vi "Input Dynamic Data Types.vi"(1 "Data Types":T2(array[cluster]), 2 "Data Names&Defaults":string[][](array[string])) -> (0 "Data Names&Data":string[][](array[string]))   [LabVIEW 2016, in "TSPopup.lvlib"]
doc: "Demo showing dynamically changing data types and working with a tree.\n\nType Sensitive Popup \nCopyright © 2007, J. David Saunders\nAll rights reserved."
uses:
  <userlib>/TSPopup/TSPopup.lvlib
  <userlib>/TSPopup/TSPopup.Popup Cluster.ctl
  <userlib>/TSPopup/TSPopup.lvclass
  <userlib>/TSPopup/TSPopup.Popup Call Parameters.ctl
  <userlib>/TSPopup/TSPopup.Data Type.ctl
panel:
  in  "Popups":T1 {"Boolean" items=["False", "True"]; "Ring" items=["X", "Y", "Z", "R1", "R3"]}
  in  "Cancel Button":bool
  in  "OK Button":bool
  in  "Data List":i32(listbox)
  # "Type Sensitive Popup \nCopyright © 2007, J. David Saunders\nAll rights reserved."
  # "Type Sensitive\nPopup"
  # "Boolean Colors"
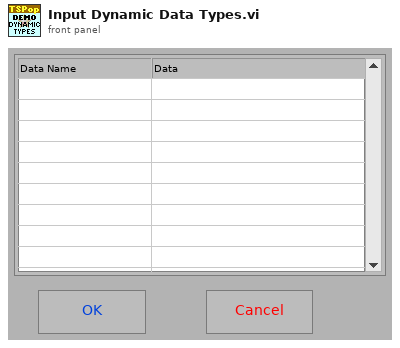
[diagram p1: front panel]
types:
  T1 = typedef "TSPopup.lvlib/TSPopup.lvclass/TSPopup.Popup Cluster.ctl" = cluster{"Unknown":bool, "Unknown 2":bool, "String":string, "Integer":i32, "Float":dbl, "Color":u32, "Boolean":u32, "Ring":u32, "Captioned String":cluster{"String":string, "OK":bool, "Cancel":bool}, "Captioned Integer":cluster{"First":i32, "OK":bool, "Cancel":bool}, "Boolean Colors":cluster{"False":cluster{"FG":u32, "BG":u32}, "True":cluster{"FG":u32, "BG":u32}, "T  to  F":cluster{"FG":u32, "BG":u32}, "F  to  T":cluster{"FG":u32, "BG":u32}, "OK":bool, "Cancel":bool}, "2-Int Cluster":cluster{"First":i32, "Second":i32, "OK":bool, "Cancel":bool}, "4-Int Cluster":cluster{"First":i32, "Second":i32, "Third":i32, "Fourth":i32, "OK":bool, "Cancel":bool}, "check":bool}
  T2 = cluster{"Data Type":string, "Caption/Ring Strings":string[]}[]
  T3 = typedef "TSPopup.lvlib/TSPopup.lvclass/TSPopup.Popup Call Parameters.ctl" = cluster{"Prop Type":T4, "Initial Value":variant, "Caption Strings":string[], "Ring Strings":string[], "Cell Rect":cluster{"left":i16, "top":i16, "right":i16, "bottom":i16}, "Mouse Coords":cluster{"x":i16, "y":i16}, "Call Data":variant}
  T4 = typedef "TSPopup.lvlib/TSPopup.lvclass/TSPopup.Data Type.ctl" = enum16{"Unkown", "NO POPUP", "String", "Integer", "Float", "Color", "Boolean", "Ring", "Captioned String", "Captioned Integer", "Button Color", "2 Int Cluster", "4 Int Cluster", "check"}
  T5 = typedef "LVPoint32TypeDef.ctl" = cluster{"Horizontal":i32, "Vertical":i32}
  T6 = typedef "TSPopup.lvlib/TSPopup.lvclass/TSPopup.Grid.Cell Info.ctl" = cluster{"Tag":string, "Row":i32, "Column":i32, "In Symbol?":bool, "In Data?":bool, "Cell String":string, "Ctl Refnum":refnum<vi>, "Prop Type":T4, "Ring Strings":string[]}
  T7 = cluster{"Data Type":string, "Caption/Ring Strings":string[]}
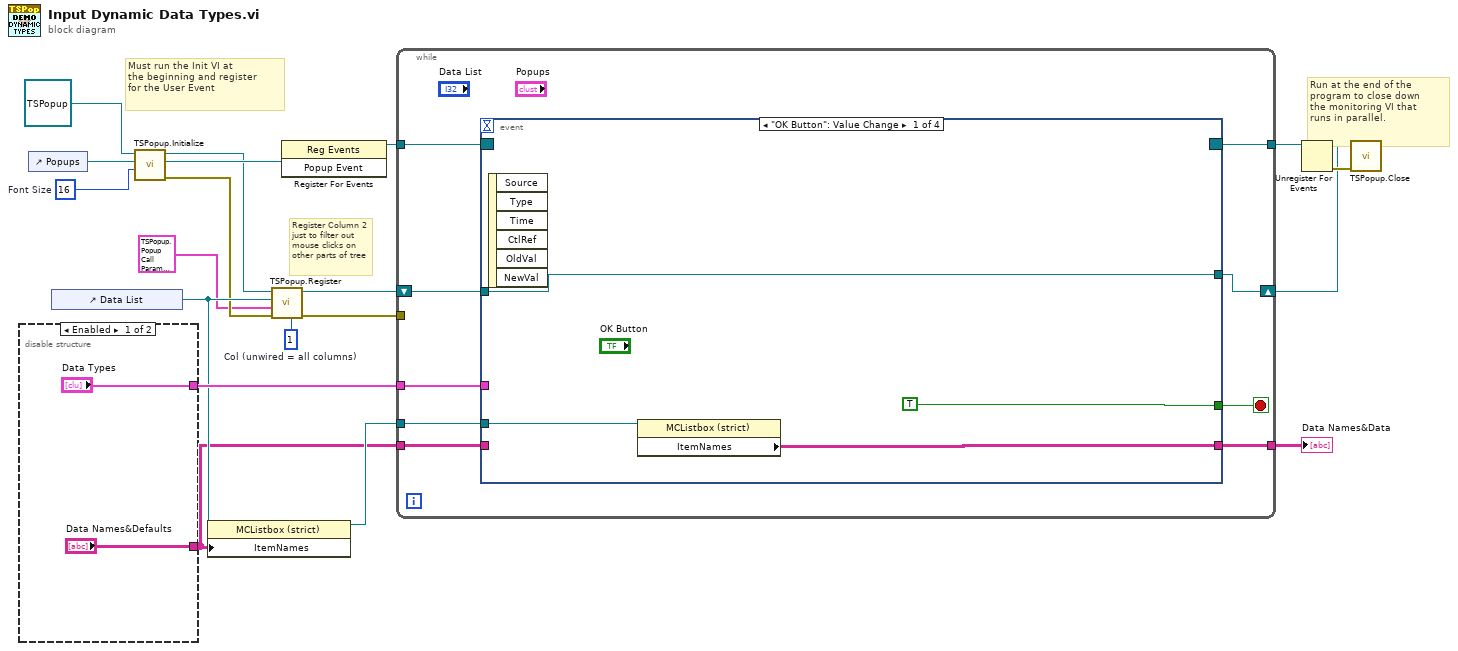
[diagram p0: block diagram]
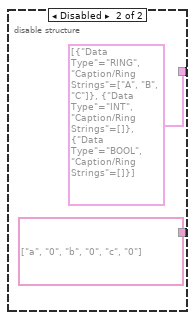
[diagram p2: hidden frame]
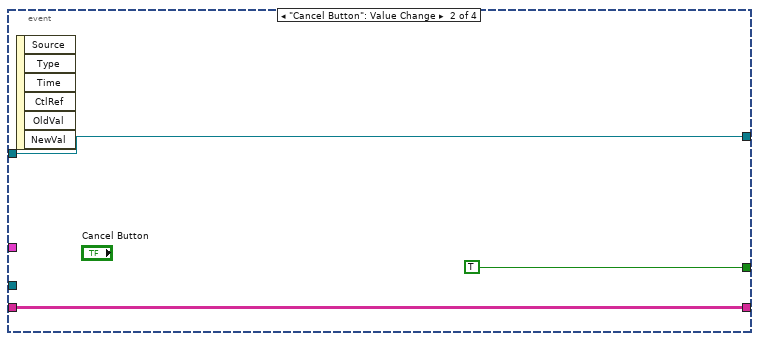
[diagram p3: hidden frame]
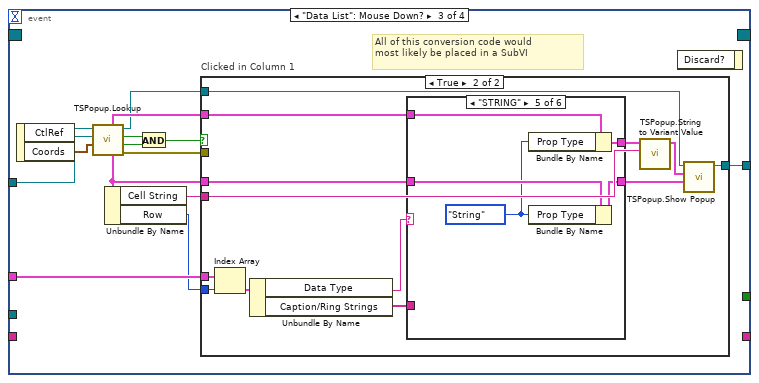
[diagram p4: hidden frame]
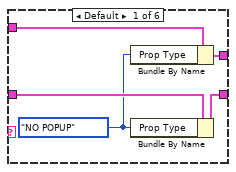
[diagram p6: hidden frame]
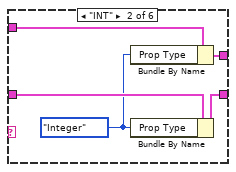
[diagram p7: hidden frame]
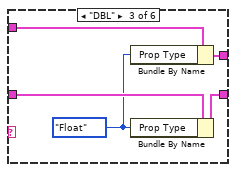
[diagram p8: hidden frame]
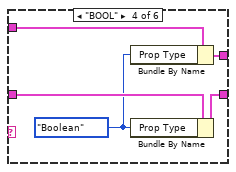
[diagram p9: hidden frame]
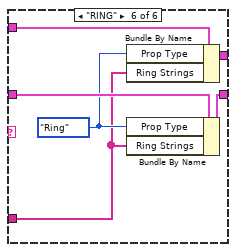
[diagram p10: hidden frame]
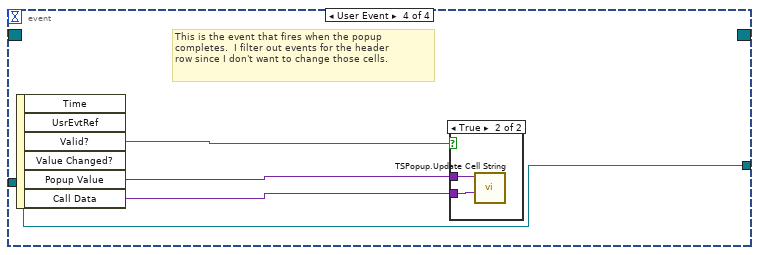
[diagram p11: hidden frame]
diagram:
  w10 = 1  # Col (unwired = all columns)
  w14 = u32 16  # Font Size
  # "Register Column 2\njust to filter out\nmouse clicks on\nother parts of tree"
  # "Run at the end of the\nprogram to close down\nthe monitoring VI that\nruns in parallel."
  # "Must run the Init VI at\nthe beginning and register\nfor the User Event"
  n1 = disable-structure shown="Enabled" {
    disable-tunnel: ["Data Types" T2 [{"Data Type"="RING", "Caption/Ring Strings"=["A", "B", "C"]}, {"Data Type"="INT", "Caption/Ring Strings"=[]}, {"Data Type"="BOOL", "Caption/Ring Strings"=[]}] ("Data Types")] -> w16
    disable-tunnel: ["Data Names&Defaults" string[][] [["a", "0"], ["b", "0"], ["c", "0"]] ("Data Names&Defaults")] -> w1
    frame Enabled {
    }
    frame Disabled {
    }
  }
  n2 = control-ref of="Popups"() -> (w4:refnum<vi>)
  n3 = control-ref of="Data List"() -> (w11:refnum<vi>)
  n4 = call <userlib>:"TSPopup.Initialize.vi"("Font Size"=w14, "Popup Cluster Ref"=w4, "TSPopup in"=refnum<class "TSPopup.lvclass"> refnum ("TSPopup.lvclass")) -> ("error out"=w8:errorcluster, "Popup Event"=w13:refnum<user-event>, "TSPopup out"=w12:refnum<class "TSPopup.lvclass">)  [unwired: 6 in]
  n5 = property class="MCListbox (strict)"(reference=w11, "ItemNames"=w1) -> (reference out=w3:refnum<vi>)  [unwired: 1 in, 1 out]
  n6 = call <userlib>:"TSPopup.Register.vi"("Col (unwired = all columns)"=w10, "error in (no error)"=w8, "Parameters"=T3 {"Prop Type"=enum."String", "Initial Value"=variant, "Caption Strings"=[], "Ring Strings"=[], "Cell Rect"={"left"=0, "top"=0, "right"=0, "bottom"=0}, "Mouse Coords"={"x"=0, "y"=0}, "Call Data"=variant}, "Ctl Refnum"=w11, "TSPopup in"=w12) -> ("error out"=w9:errorcluster, "TSPopup out"=w7:refnum<class "TSPopup.lvclass">)  [unwired: 4 in, 1 out]
  n7 = register-events(w13) -> (reference out=w19:refnum<event-registration>)  [unwired: 2 in, 1 out]
  n8 = while {
    tunnel: w19 -> [w32]
    tunnel: [w31] -> w18
    tunnel: w16 -> [w29]
    tunnel: w9 -> [_]
    shift-right: [w27] -> w6
    shift-left: w7 -> [w28]
    tunnel: w3 -> [w26]
    tunnel: [w25] -> w2
    tunnel: w1 -> [w24]
    stop <- w30 stop-if-true
    n9 = event shown="[0] \"OK Button\": Value Change" {
      selector: w32 -> [_ _ _ _]
      dyn-events: [_ _ _ _] -> w31
      timeout: _ -> [_ _ _ _]
      tunnel: [TRUE TRUE _ _] -> w30
      tunnel: w29 -> [_ _ w51 _]
      tunnel: w28 -> [w35 w38 w42 w99]
      tunnel: [w35 w38 w40 w99] -> w27
      tunnel: w26 -> [w34 _ _ _]
      tunnel: [w33 w37 _ _] -> w25
      tunnel: w24 -> [_ w37 _ _]
      event "OK Button": Value Change {
        n10 = event-data() -> ()  [unwired: 1 in, 6 out]
        n11 = property class="MCListbox (strict)"(reference=w34) -> ("ItemNames"=w33:string[][])  [unwired: 1 in, 2 out]
      }
      event "Cancel Button": Value Change {
        n12 = event-data() -> ()  [unwired: 1 in, 6 out]
      }
      event "Data List": Mouse Down? {
        # "All of this conversion code would\nmost likely be placed in a SubVI"
        n13 = event-data() -> ("CtlRef"=w49:refnum<vi>, "Coords"=w48:T5)  [unwired: 1 in]
        n14 = call <userlib>:"TSPopup.Lookup.vi"("Point"=w48, "Ctl Refnum"=w49, "TSPopup in"=w42) -> ("error out"=w44:errorcluster, "In Bounds?"=w45:bool, "Found"=w46:bool, "TSPopup out"=w41:refnum<class "TSPopup.lvclass">, "Cell Info (Call data)"=w43:T6, "Popup Parameters"=w47:T3)  [unwired: 3 in]
        n15 = Unbundle By Name(w43) -> ("Cell String"=w52:string, "Row"=w50:i32)
        n16 = And(x=w46, y=w45) -> (x .and. y?=w53:bool)
        n17 = case "Clicked in Column 1" shown="True" w53 {
          tunnel: w47 -> [_ w67]
          tunnel: w43 -> [_ w66]
          tunnel: w44 -> [_ _]
          tunnel: w52 -> [_ w64]
          tunnel: w51 -> [_ w61]
          tunnel: w50 -> [_ w60]
          tunnel: w41 -> [w54 w56]
          tunnel: [w54 w55] -> w40
          frame False {
          }
          frame True {
            n18 = Index Array(array=w61, index=w60) -> (element=w59:T7)
            n19 = Unbundle By Name(w59) -> ("Data Type"=w58:string, "Caption/Ring Strings"=w57:string[])
            n20 = case shown="\"STRING\"" w58 {
              tunnel: w67 -> [w72 w77 w82 w87 w92 w98]
              tunnel: w66 -> [w71 w76 w81 w86 w91 w97]
              tunnel: [w70 w75 w80 w85 w90 w96] -> w65
              tunnel: [w68 w73 w78 w83 w88 w94] -> w62
              tunnel: w57 -> [_ _ _ _ _ w93]
              frame Default {
                w69 = TSPopup.Data_Type."NO POPUP"
                n21 = Bundle By Name(cluster=w72, "Prop Type"=w69) -> (w68:T3)
                n22 = Bundle By Name(cluster=w71, "Prop Type"=w69) -> (w70:T6)
              }
              frame "INT" {
                w74 = TSPopup.Data_Type."Integer"
                n23 = Bundle By Name(cluster=w77, "Prop Type"=w74) -> (w73:T3)
                n24 = Bundle By Name(cluster=w76, "Prop Type"=w74) -> (w75:T6)
              }
              frame "DBL" {
                w79 = TSPopup.Data_Type."Float"
                n25 = Bundle By Name(cluster=w82, "Prop Type"=w79) -> (w78:T3)
                n26 = Bundle By Name(cluster=w81, "Prop Type"=w79) -> (w80:T6)
              }
              frame "BOOL" {
                w84 = TSPopup.Data_Type."Boolean"
                n27 = Bundle By Name(cluster=w87, "Prop Type"=w84) -> (w83:T3)
                n28 = Bundle By Name(cluster=w86, "Prop Type"=w84) -> (w85:T6)
              }
              frame "STRING" {
                w89 = TSPopup.Data_Type."String"
                n29 = Bundle By Name(cluster=w92, "Prop Type"=w89) -> (w88:T3)
                n30 = Bundle By Name(cluster=w91, "Prop Type"=w89) -> (w90:T6)
              }
              frame "RING" {
                w95 = TSPopup.Data_Type."Ring"
                n31 = Bundle By Name(cluster=w98, "Prop Type"=w95, "Ring Strings"=w93) -> (w94:T3)
                n32 = Bundle By Name(cluster=w97, "Prop Type"=w95, "Ring Strings"=w93) -> (w96:T6)
              }
            }
            n33 = call <userlib>:"TSPopup.String to Variant Value.vi"("Cell String"=w64, "Popup Parameters"=w62) -> ("Popup Parameters out"=w63:T3)  [unwired: 7 in, 2 out]
            n34 = call <userlib>:"TSPopup.Show Popup.vi"("Call Data (ignore if empty)"=w65, "Popup Parameters"=w63, "TSPopup in"=w56) -> ("TSPopup out"=w55:refnum<class "TSPopup.lvclass">)  [unwired: 7 in, 1 out]
          }
        }
        n35 = event-data() -> ()  [unwired: 2 in, 1 out]
      }
      event User Event {
        # "This is the event that fires when the popup\ncompletes.  I filter out events for the header\nrow since I don't want to change those cells."
        n36 = event-data() -> ("Valid?"=w102:bool, "Popup Value"=w101:variant, "Call Data"=w100:variant)  [unwired: 1 in, 3 out]
        n37 = case shown="True" w102 {
          tunnel: w101 -> [_ w103]
          tunnel: w100 -> [_ w104]
          frame False {
          }
          frame True {
            n38 = call <userlib>:"TSPopup.Update Cell String.vi"("Call Data (must be Cell Info cluster)"=w104, "Popup Value"=w103) -> ()  [unwired: 9 in, 1 out]
          }
        }
      }
    }
  }
  "Data Names&Data" <- w2
  n39 = Unregister For Events(event registration refnum=w18) -> (error out=w17:errorcluster)  [unwired: 1 in]
  n40 = call <userlib>:"TSPopup.Close.vi"("error in (no error)"=w17, "TSPopup in"=w6) -> ()  [unwired: 8 in, 2 out]
